vi "Set Initialization Data - AppMgr.vi"(8 "error in":errorcluster, 11 "Debug Server in":refnum<class "Debug Server.lvclass">) -> (0 "error out":errorcluster, 3 "Debug Server out":refnum<class "Debug Server.lvclass">)   [LabVIEW 2017, in "Debug Server.lvclass"]
doc: "Sets the initialization data of a statically linked subWorker."
uses:
  Debug Server.lvclass
  Application Manager/Initialization Data.ctl
  Application Manager/Response Cases.ctl
  <vilib>/addons/_Workers/Library/Case Label.ctl
  Debug Server.lvclass/Debug Server.ctl
  Application Manager/Application Manager.lvclass
  C:/Program Files (x86)/National Instruments/LabVIEW 2017/vi.lib/addons/_Workers/Library/Classes/Worker/Worker.lvclass
  <vilib>/addons/_Workers/Library/Workers.lvlib
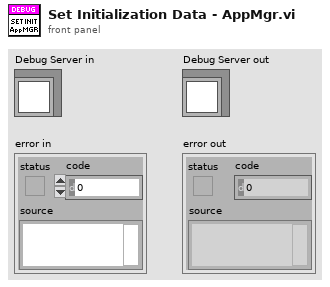
[diagram p1: front panel]
types:
  T1 = typedef "Application Manager.lvclass/Initialization Data.ctl" = cluster{"Response Cases":T2}
  T2 = typedef "Application Manager.lvclass/Response Cases.ctl" = cluster{"Show Settings Dialog":T3, "Start Shutdown":T3, "Show Message Log":T3, "New Head Worker Added":T3, "Show Worker Front Panel":T3, "Show Worker Block Diagram":T3, "Send Start Exiting Request":T3, "Filter as Enque Worker":T3, "Filter as Deque Worker":T3, "Go to MHL Case - Response":T3}
  T3 = typedef "Workers.lvlib/Case Label.ctl" = string
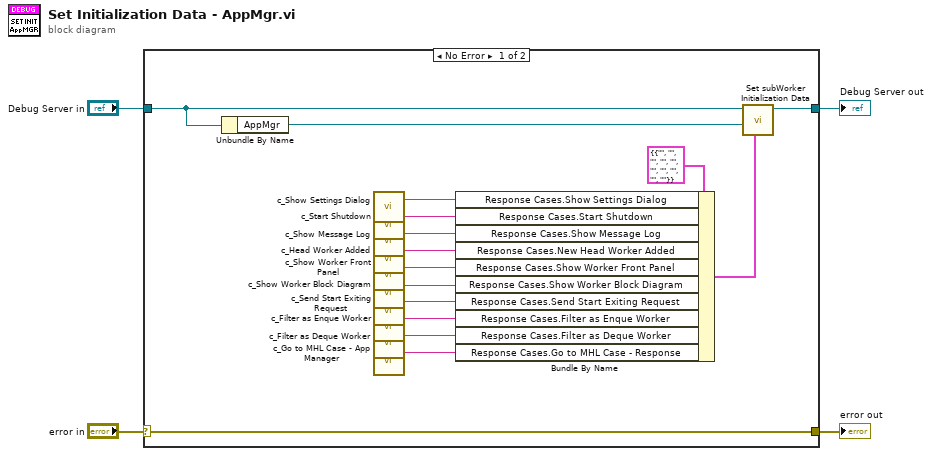
[diagram p0: block diagram]
diagram:
  n1 = case shown="No Error" "error in" {
    selector: "error in" -> [w20 w22]
    tunnel: [w20 w22] -> w3
    tunnel: [w18 w21] -> w2
    tunnel: "Debug Server in" -> [w17 w21]
    frame No Error {
      n2 = Unbundle By Name(w17) -> ("AppMgr"=w19:refnum<class "Application Manager.lvclass">)
      n3 = call "c_Show Settings Dialog.vi"() -> ("Case Label"=w14:T3)  [unwired: 1 in]
      n4 = call "c_Start Shutdown.vi"() -> ("Case Label"=w13:T3)  [unwired: 1 in]
      n5 = call "c_Show Message Log.vi"() -> ("Case Label"=w12:T3)  [unwired: 1 in]
      n6 = call "c_Head Worker Added.vi"() -> ("Case Label"=w11:T3)  [unwired: 1 in]
      n7 = call "c_Show Worker Front Panel.vi"() -> ("Case Label"=w10:T3)  [unwired: 1 in]
      n8 = call "c_Show Worker Block Diagram.vi"() -> ("Case Label"=w9:T3)  [unwired: 1 in]
      n9 = call "c_Send Start Exiting Request.vi"() -> ("Case Label"=w8:T3)  [unwired: 1 in]
      n10 = call "c_Filter as Enque Worker.vi"() -> ("Case Label"=w7:T3)  [unwired: 1 in]
      n11 = call "c_Filter as Deque Worker.vi"() -> ("Case Label"=w6:T3)  [unwired: 1 in]
      n12 = call "c_Go to MHL Case - App Manager.vi"() -> ("Case Label"=w5:T3)  [unwired: 1 in]
      n13 = Bundle By Name(cluster=T1 {"Response Cases"={"Show Settings Dialog"="", "Start Shutdown"="", "Show Message Log"="", "New Head Worker Added"="", "Show Worker Front Panel"="", "Show Worker Block Diagram"="", "Send Start Exiting Request"="", "Filter as Enque Worker"="", "Filter as Deque Worker"="", "Go to MHL Case - Response"=""}} ("Initialization Data"), "Response Cases.Show Settings Dialog"=w14, "Response Cases.Start Shutdown"=w13, "Response Cases.Show Message Log"=w12, "Response Cases.New Head Worker Added"=w11, "Response Cases.Show Worker Front Panel"=w10, "Response Cases.Show Worker Block Diagram"=w9, "Response Cases.Send Start Exiting Request"=w8, "Response Cases.Filter as Enque Worker"=w7, "Response Cases.Filter as Deque Worker"=w6, "Response Cases.Go to MHL Case - Response"=w5) -> (w15:T1)
      n14 = call-dynamic "Set subWorker Initialization Data.vi"("Initialization Data"=w15, "subWorker"=w19, "Worker"=w17) -> ("Worker out"=w18:refnum<class "Debug Server.lvclass">)  [unwired: 8 in]
    }
    frame Error {
    }
  }
  "error out" <- w3
  "Debug Server out" <- w2
